vi "Client.vi"() -> ()   [LabVIEW 2015]
doc: "This VI implements a client for the TCP Named Service - Server.vi. It connects to a service by specifying the server address and the name of the service. The client receives the string sent by the server, displays the string and closes the connection."
panel:
  in  "stop":bool
  out "Message from Server":string
  # "Overview: Demonstrates the use of the TCP functions to connect to a TCP server VI via named service and receive data.\nInstructions:\n1. Ensure TCP Named Service - Server.vi is already running.\n2. Run the VI."
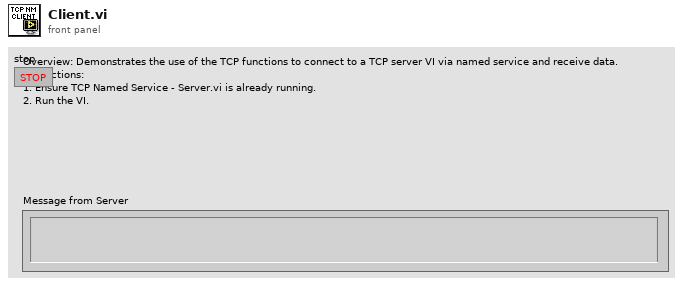
[diagram p1: front panel]
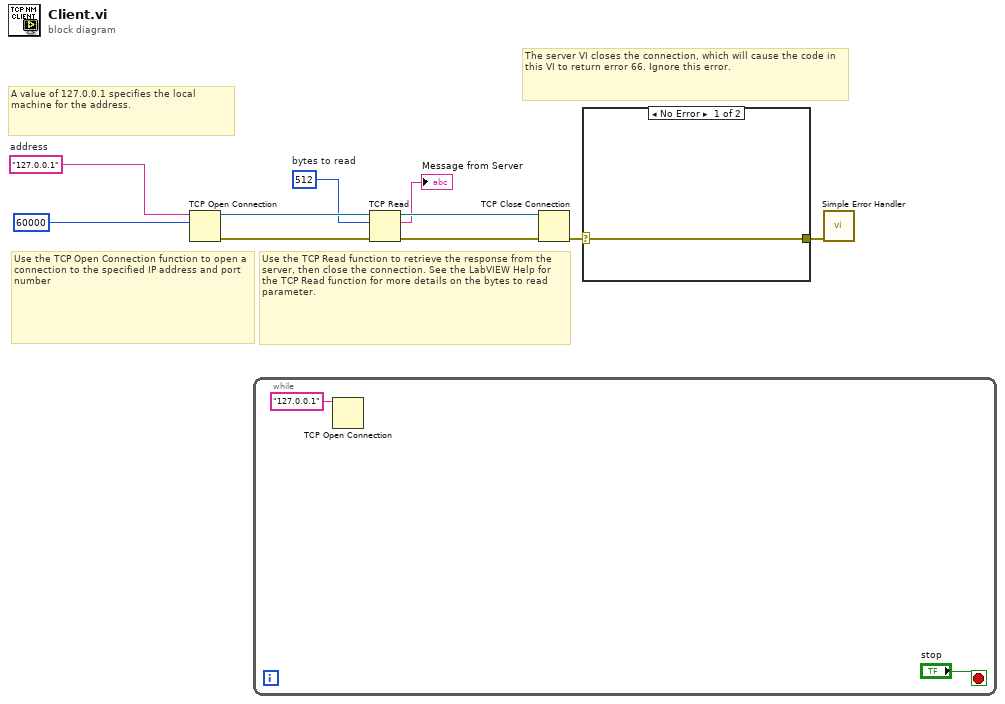
[diagram p0: block diagram]
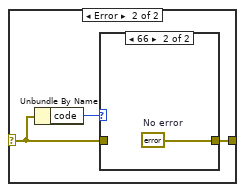
[diagram p2: hidden frame]
diagram:
  w4 = 512  # bytes to read
  w5 = "127.0.0.1"  # address
  # "The server VI closes the connection, which will cause the code in this VI to return error 66. Ignore this error."
  # "A value of 127.0.0.1 specifies the local machine for the address."
  # "Use the TCP Open Connection function to open a connection to the specified IP address and port number"
  # "Use the TCP Read function to retrieve the response from the server, then close the connection. See the LabVIEW Help for the TCP Read function for more details on the bytes to read parameter."
  n1 = TCP Open Connection(address=w5, remote port or service name=u16 60000) -> (connection ID=w9:refnum<k5>, error out=w10:errorcluster)  [unwired: 3 in]
  n2 = while {
    stop <- "stop" stop-if-true
    n3 = TCP Open Connection(address="127.0.0.1") -> ()  [unwired: 4 in, 2 out]
  }
  n4 = TCP Read(connection ID=w9, bytes to read=w4, error in (no error)=w10) -> (connection ID out=w8:refnum<k5>, data out=→"Message from Server":string, error out=w7:errorcluster)  [unwired: 2 in]
  n5 = TCP Close Connection(connection ID=w8, error in (no error)=w7) -> (error out=w3:errorcluster)  [unwired: 1 in, 1 out]
  n6 = case shown="No Error" w3 {
    selector: w3 -> [w13 w15]
    tunnel: [w13 w14] -> w2
    frame No Error {
    }
    frame Error {
      n7 = Unbundle By Name(w15) -> ("code"=w16:i32)
      n8 = case shown="66" w16 {
        tunnel: w15 -> [w17 _]
        tunnel: [w17 w18] -> w14
        frame Default {
        }
        frame 66 {
          w18 = errorcluster {"status"=FALSE, "code"=0, "source"=""}  # No error
        }
      }
    }
  }
  n9 = call <vilib>:"Simple Error Handler.vi"("error in (no error)"=w2) -> ()  [unwired: 4 in, 5 out]
